vi "CRYAna 2Ch Nb FFT.vi"(8 "Wave Size (Sp)":i32=100000, 9 "Overlap (%)":dbl, 10 "dF(Hz)":dbl=10.0, 11 "Fs(Hz)":dbl=44100.0) -> (0 "Increment (Sp)":i32, 1 "New dF (Hz)":dbl, 2 "#FFT's(-)":i32, 3 "FFT Size(Sp)":i32)   [LabVIEW 2013]
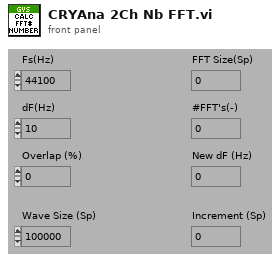
[diagram p1: front panel]
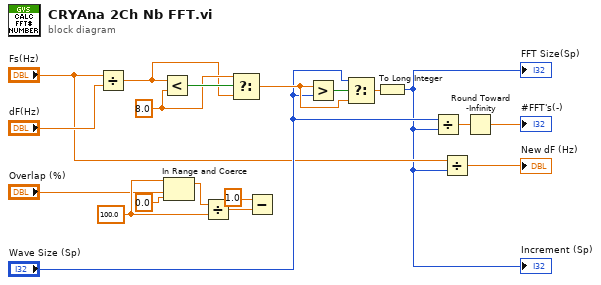
[diagram p0: block diagram]
diagram:
  w3 = 100.0 ("upper limit")
  w17 = 8.0 ("y")
  n1 = Divide(x="Fs(Hz)", y="dF(Hz)") -> (x/y=w13:dbl)
  n2 = Less?(x=w13, y=w17) -> (x < y?=w18:bool)
  n3 = In Range and Coerce(upper limit=w3, x="Overlap (%)", lower limit=0.0) -> (coerced(x)=w4:dbl)  [unwired: 1 out]
  n4 = Divide(x=w4, y=w3) -> (x/y=w2:dbl)
  n5 = Select(t=w17, s=w18, f=w13) -> (s? t:f=w15:dbl)
  n6 = Subtract(x=1.0, y=w2) -> ()  [unwired: 1 out]
  n7 = Greater?(x=w15, y="Wave Size (Sp)") -> (0:w16:bool)
  n8 = Select(t="Wave Size (Sp)", s=w16, f=w15) -> (s? t:f=w14:dbl)
  n9 = To Long Integer(number=w14) -> (32bit integer=w8:i32)
  "FFT Size(Sp)" <- w8
  "Increment (Sp)" <- w8
  n10 = Divide(x="Wave Size (Sp)", y=w8) -> (x/y=w11:dbl)
  n11 = Divide(x="Fs(Hz)", y=w8) -> (x/y=→"New dF (Hz)":dbl)
  n12 = Round Toward -Infinity(1:w11) -> (0:→"#FFT's(-)":dbl)
